vi "Untitled 1.vi"() -> ()   [LabVIEW 2020]
panel:
  in  "Numeric 3":dbl
  out "Numeric 2":i32
  in  "°F 2":dbl(slide) scale=0.0..150.0
  out "x*y 2":dbl
  out "°C 2":dbl(slide) scale=0.0..100.0
  in  "stop 2":bool
  in  "Boolean 2":bool
  out "Numeric":i32
  out "°C":dbl(slide) scale=0.0..100.0
  out "x*y":dbl
  in  "°F":dbl(slide) scale=0.0..150.0
  in  "stop":bool
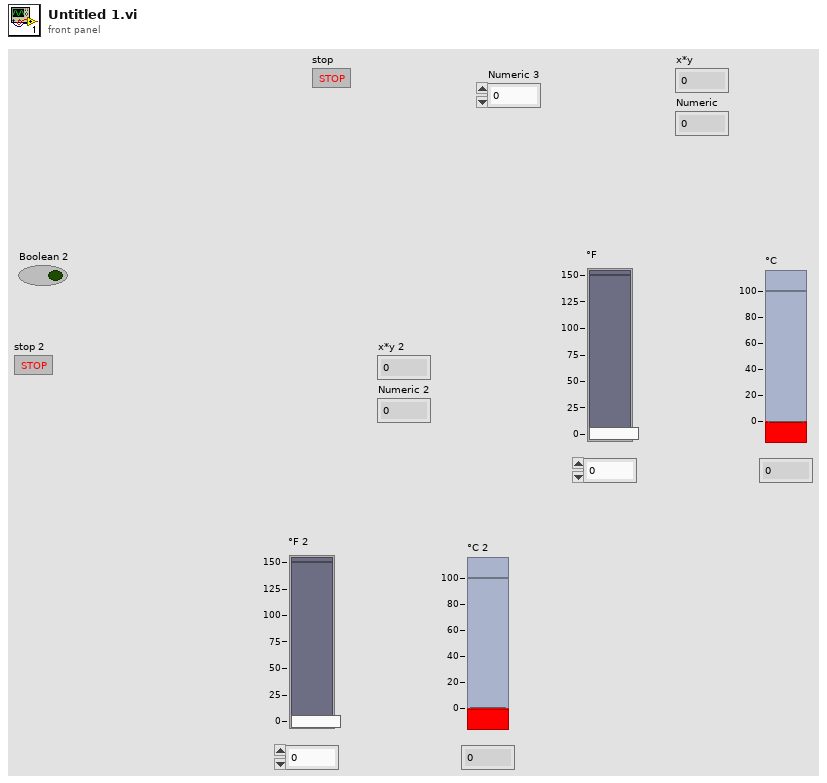
[diagram p1: front panel]
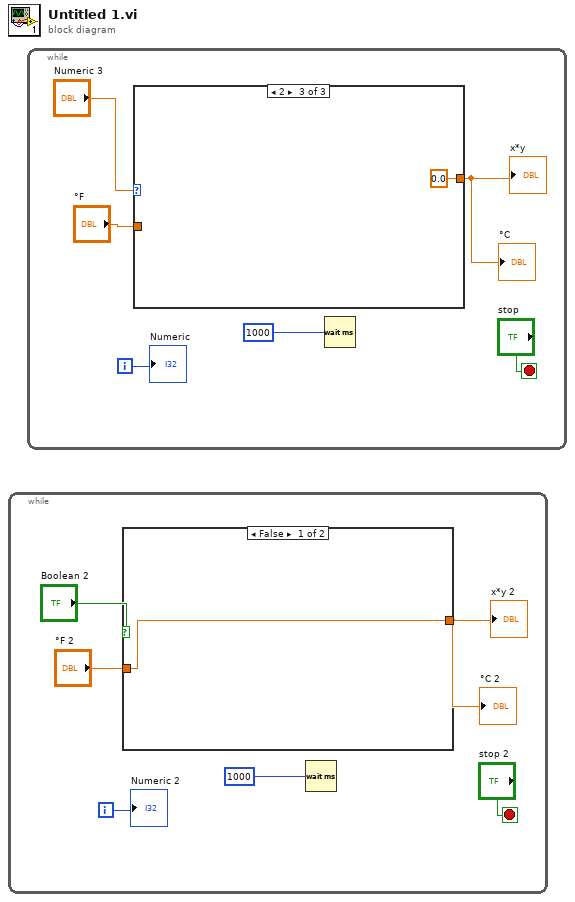
[diagram p0: block diagram]
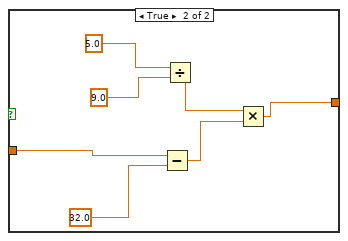
[diagram p2: hidden frame]
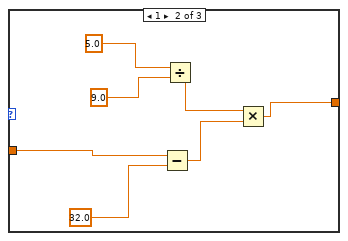
[diagram p4: hidden frame]
diagram:
  n1 = while {
    i -> [w6]
    stop <- "stop 2" stop-if-true
    n2 = case shown="False" "Boolean 2" {
      tunnel: [w7 w9] -> w4
      tunnel: "°F 2" -> [w7 w8]
      frame False {
      }
      frame True {
        n3 = Subtract(x=w8, y=32.0) -> (x-y=w10:dbl)
        n4 = Divide(x=5.0, y=9.0) -> (x/y=w11:dbl)
        n5 = Multiply(x=w11, y=w10) -> (x*y=w9:dbl)
      }
    }
    "x*y 2" <- w4
    "°C 2" <- w4
    n6 = Wait (ms)(milliseconds to wait=u32 1000) -> ()  [unwired: 1 out]
    "Numeric 2" <- w6
  }
  n7 = while {
    i -> [w20]
    stop <- "stop" stop-if-true
    n8 = case shown="2" "Numeric 3" {
      tunnel: [w21 w23 0.0 ("°F")] -> w18
      tunnel: "°F" -> [w21 w22 _]
      frame 0, Default {
      }
      frame 1 {
        n9 = Subtract(x=w22, y=32.0) -> (x-y=w24:dbl)
        n10 = Divide(x=5.0, y=9.0) -> (x/y=w25:dbl)
        n11 = Multiply(x=w25, y=w24) -> (x*y=w23:dbl)
      }
      frame 2 {
      }
    }
    "x*y" <- w18
    "°C" <- w18
    n12 = Wait (ms)(milliseconds to wait=u32 1000) -> ()  [unwired: 1 out]
    "Numeric" <- w20
  }
